vi "Check Package.vi"(8 "error in (no error)":errorcluster, 10 "Package":refnum<class "PackageAbstract.lvclass">, 11 "InitAction in":refnum<class "InitAction.lvclass">) -> (0 "error out":errorcluster, 2 "Problems":string[](array[string]), 3 "InitAction out":refnum<class "InitAction.lvclass">)   [LabVIEW 2020, in "GPackTools.lvlib" / "InitAction.lvclass"]
uses:
  InitAction.lvclass
  GPack/PackageAbstract/PackageAbstract.lvclass
  InitAction.lvclass/InitAction.ctl
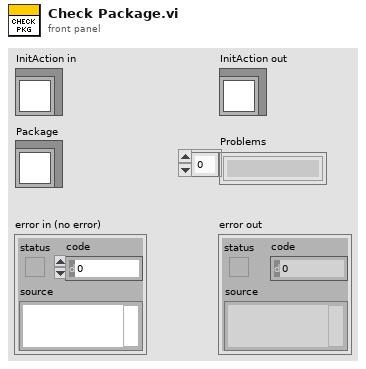
[diagram p1: front panel]
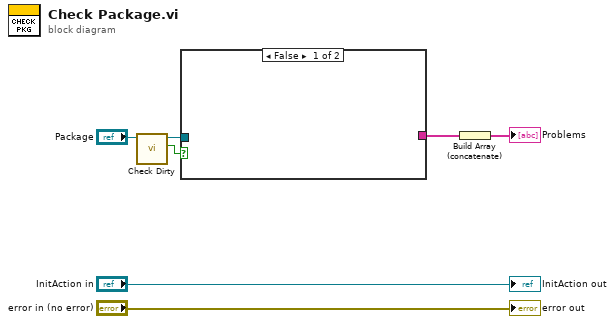
[diagram p0: block diagram]
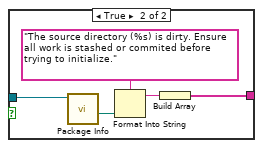
[diagram p2: hidden frame]
diagram:
  n1 = call-dynamic "Check Dirty.vi"("Package in"="Package") -> ("Dirty"=w4:bool, "Package out"=w3:refnum<class "PackageAbstract.lvclass">)  [unwired: 8 in, 1 out]
  n2 = case shown="False" w4 {
    tunnel: w3 -> [_ w11]
    tunnel: [_ w8] -> w2
    frame False {
    }
    frame True {
      n3 = call-dynamic "Package Info.vi"("Package in"=w11) -> ("Folder"=w10:path)  [unwired: 8 in, 2 out]
      n4 = Format Into String(format string="The source directory (%s) is dirty. Ensure all work is stashed or commited before trying to initialize.", w10) -> (resulting string=w9:string)  [unwired: 2 in, 1 out]
      n5 = Build Array(w9) -> (w8:string[])
    }
  }
  n6 = Build Array (concatenate)(w2) -> (→"Problems":string[])
  "error out" <- "error in (no error)"
  "InitAction out" <- "InitAction in"
